vi "macro_TrapezoidProfile_Execute.vi"   [LabVIEW 2019, in "Trajectory_Library.lvlib"]
uses:
  Trajectory_Library.lvlib
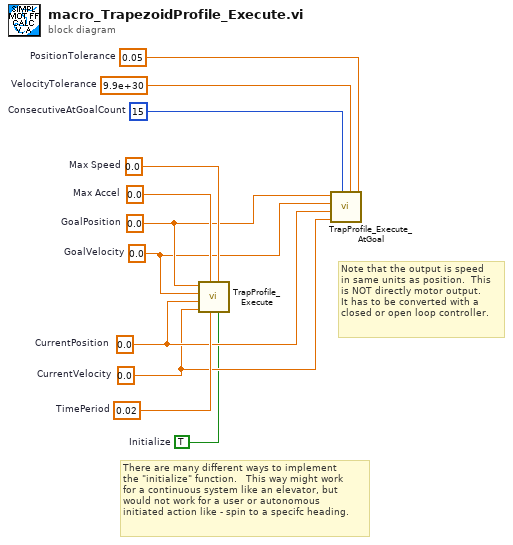
[diagram p0: block diagram]
diagram:
  w6 = 15  # ConsecutiveAtGoalCount
  w7 = 9.9e+30  # VelocityTolerance
  w8 = 0.05  # PositionTolerance
  w3 = 0.0  # GoalPosition
  w2 = 0.0  # GoalVelocity
  w5 = 0.0  # CurrentPosition
  w4 = 0.0  # CurrentVelocity
  w9 = 0.0  # Max Accel
  w10 = 0.02  # TimePeriod
  w11 = 0.0  # Max Speed
  w1 = TRUE  # Initialize
  # "Note that the output is speed\nin same units as position.  This\nis NOT directly motor output.\nIt has to be converted with a \nclosed or open loop controller."
  # "There are many different ways to implement\nthe \"initialize\" function.   This way might work\nfor a continuous system like an elevator, but\nwould not work for a user or autonomous \ninitiated action like - spin to a specifc heading."
  n1 = call "TrapProfile_Execute.vi"("Initialize"=w1, "Max Speed"=w11, "TimePeriod"=w10, "Max Accel"=w9, "CurrentVelocity"=w4, "CurrentPosition"=w5, "GoalVelocity"=w2, "GoalPosition"=w3) -> ()  [unwired: 4 out]
  n2 = call "TrapProfile_Execute_AtGoal.vi"("PositionTolerance"=w8, "VelocityTolerance"=w7, "ConsecutiveAtGoalCount"=w6, "CurrentVelocity"=w4, "CurrentPosition"=w5, "GoalVelocity"=w2, "GoalPosition"=w3) -> ()  [unwired: 4 in, 1 out]
